vi "Simulator SNA Check Waveform Timing.vi"(8 "error in (no error)":errorcluster, 10 "dt":dbl=1.0, 11 "signal in":waveform(dbl)) -> (0 "error out":errorcluster, 3 "timing ok":bool=TRUE)   [LabVIEW 2011]
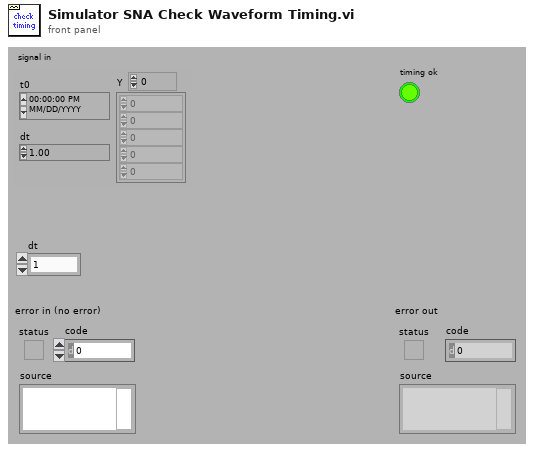
[diagram p1: front panel]
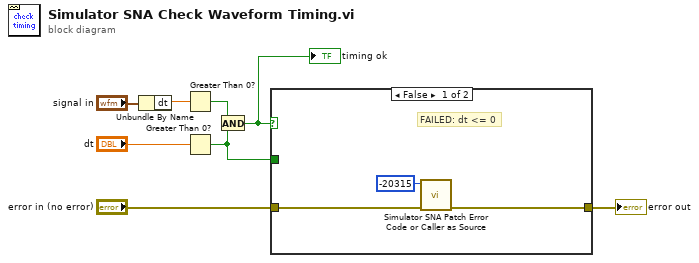
[diagram p0: block diagram]
diagram:
  n1 = Unbundle By Name("signal in") -> ("dt"=w2:dbl)
  n2 = Greater Than 0?(x=w2) -> (x > 0?=w8:bool)
  n3 = Greater Than 0?(x="dt") -> (x > 0?=w7:bool)
  n4 = And(x=w8, y=w7) -> (x .and. y?=w6:bool)
  "timing ok" <- w6
  n5 = case shown="False" w6 {
    tunnel: w7 -> [_ _]
    tunnel: "error in (no error)" -> [w11 w12]
    tunnel: [w10 w12] -> w5
    frame False {
      # "FAILED: dt <= 0"
      n6 = call "Simulator SNA Patch Error Code or Caller as Source.vi"("error in (no error)"=w11, "error code"=-20315 ("code")) -> ("error out"=w10:errorcluster)  [unwired: 2 in, 7 out]
    }
    frame True {
      # "timing ok  (dt > 0)"
    }
  }
  "error out" <- w5
